vi "WriteEdvrRef.vi"(8 "error in (no error)":errorcluster, 10 "Edvr":T1, 11 "EdvrObject in":refnum<class "EdvrObject.lvclass">) -> (0 "error out":errorcluster, 3 "EdvrObject out":refnum<class "EdvrObject.lvclass">)   [LabVIEW 2020, in "OpenLvVision_OpenCv.lvlib" / "EdvrObject.lvclass"]
uses:
  EdvrObject.lvclass
  TypeDef/Edvr.ctl
  EdvrObject.lvclass/EdvrObject.ctl
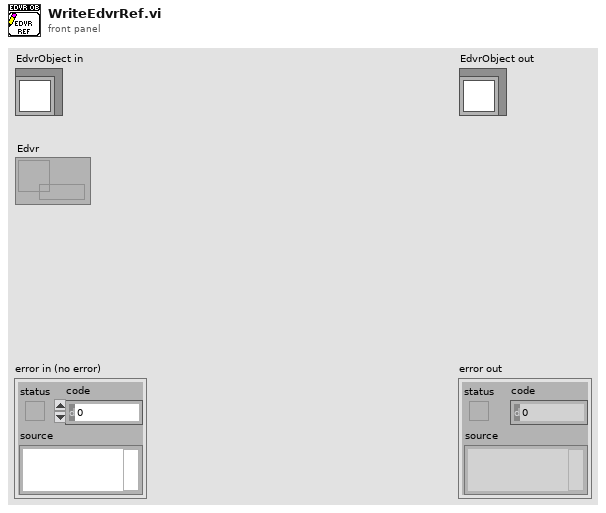
[diagram p1: front panel]
types:
  T1 = typedef "OpenLvVision_OpenCv.lvlib/EdvrObject.lvclass/Edvr.ctl" = refnum<data-value>
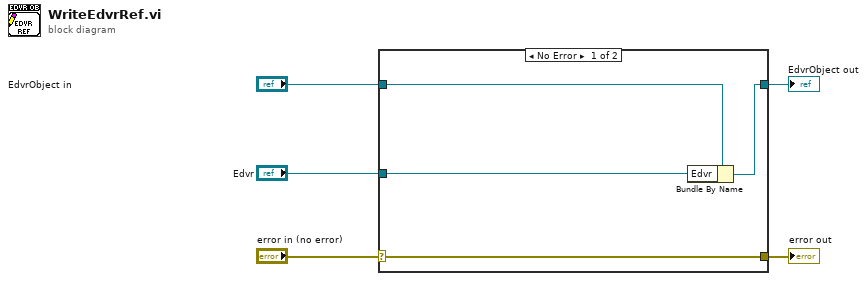
[diagram p0: block diagram]
diagram:
  n1 = case shown="No Error" "error in (no error)" {
    selector: "error in (no error)" -> [w9 w10]
    tunnel: [w9 w10] -> w4
    tunnel: [w7 w11] -> w2
    tunnel: "EdvrObject in" -> [w8 w11]
    tunnel: "Edvr" -> [w6 _]
    frame No Error {
      n2 = Bundle By Name(cluster=w8, "Edvr"=w6) -> (w7:refnum<class "EdvrObject.lvclass">)
    }
    frame Error {
    }
  }
  "error out" <- w4
  "EdvrObject out" <- w2
